vi "W7X1DPut_Reduced.vi"(4 "dimensions":i64[](array[numeric])=[1428413878000000000, -1], 7 "Unit":string="s", 9 "values":T1(array[cluster]), 10 "SigJSONbuffer":string, 11 "SigLabel":string="MTau") -> (0 "Parlog error out":errorcluster, 1 "file path written":string)   [LabVIEW 2014]
uses:
  <vilib>/httpClient/POSTBuffer.vi
  <vilib>/httpClient/LabVIEWHTTPClient.lvlib
panel:
  in  "?":T2
  out "JSON string":string
  out "body":string
  out "headers":string
  out "body Parlog":string
  out "headers parms":string
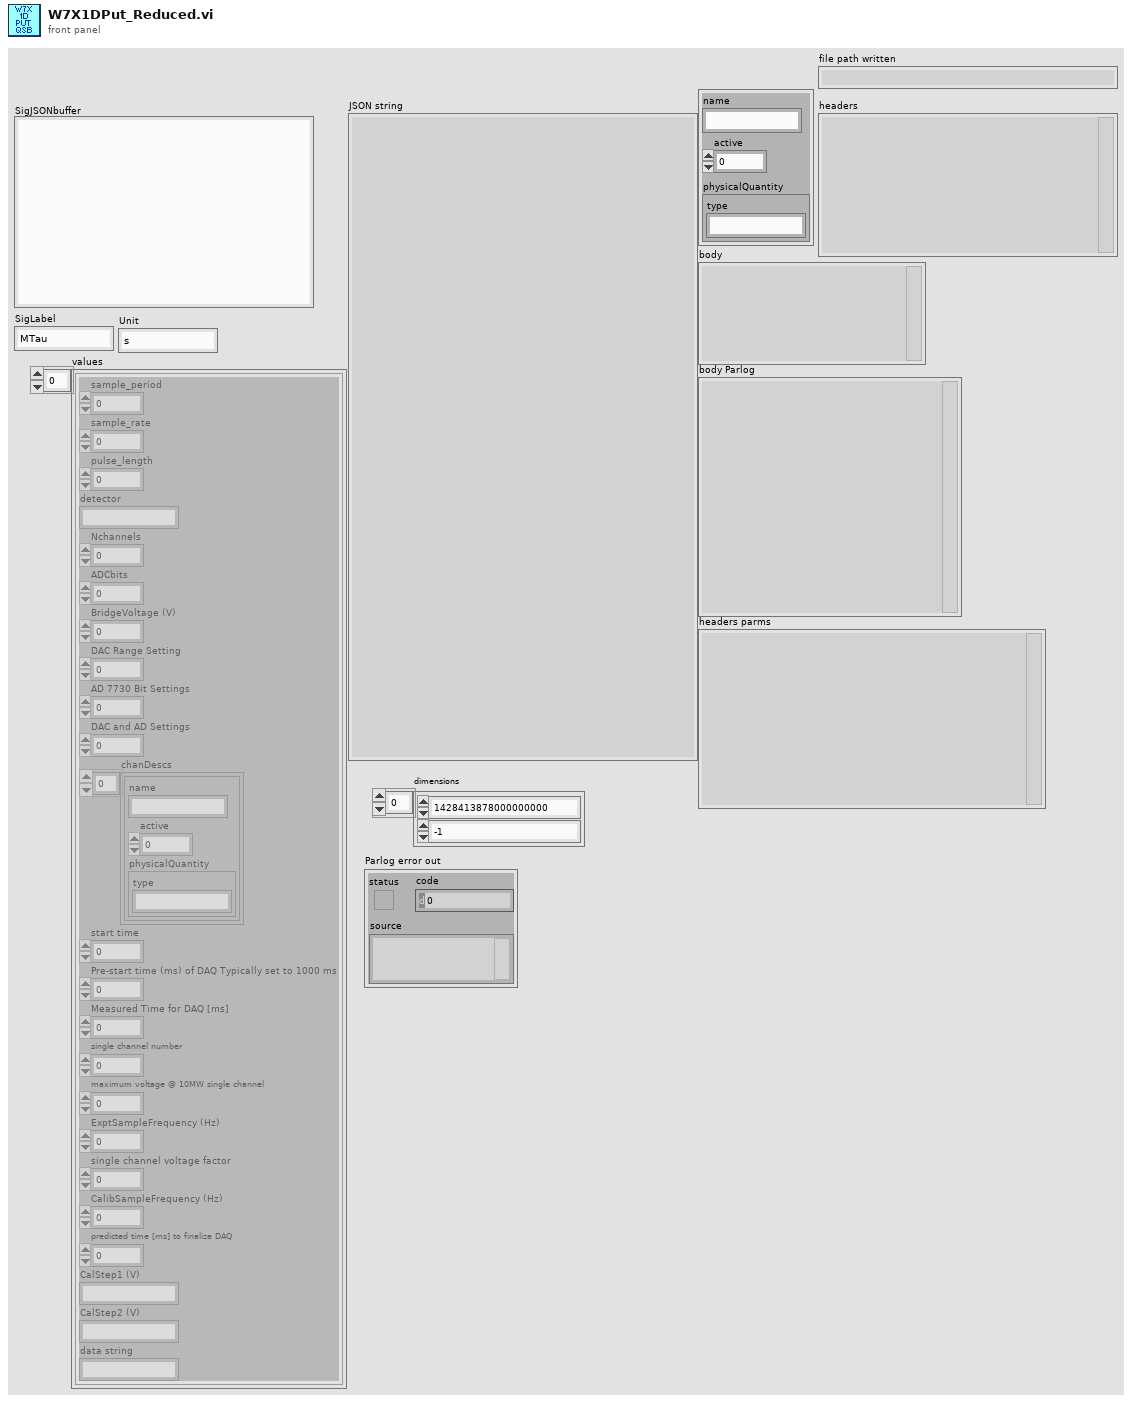
[diagram p1: front panel]
types:
  T1 = cluster{"sample_period":dbl, "sample_rate":dbl, "pulse_length":dbl, "detector":string, "Nchannels":i16, "ADCbits":i16, "BridgeVoltage (V)":sgl, "DAC Range Setting":u8, "AD 7730 Bit Settings":i32, "DAC and AD Settings":i32, "chanDescs":cluster{"name":string, "active":i32, "physicalQuantity":cluster{"type":string}}[], "start time":i64, "Pre-start time (ms) of DAQ Typically set to 1000 ms":i32, "Measured Time for DAQ [ms] ":u32, "single channel number":i64, "maximum voltage @ 10MW single channel":dbl, "ExptSampleFrequency (Hz)":sgl, "single channel voltage factor":dbl, "CalibSampleFrequency (Hz)":sgl, "predicted time [ms] to finalize DAQ":dbl, "CalStep1 (V)":string, "CalStep2 (V)":string, "data string":string}[]
  T2 = cluster{"name":string, "active":i32, "physicalQuantity":cluster{"type":string}}
  T3 = cluster{"sample_period":dbl, "sample_rate":dbl, "pulse_length":dbl, "detector":string, "Nchannels":i16, "ADCbits":i16, "BridgeVoltage (V)":sgl, "DAC Range Setting":u8, "AD 7730 Bit Settings":i32, "DAC and AD Settings":i32, "chanDescs":cluster{"name":string, "active":i32, "physicalQuantity":cluster{"type":string}}[], "start time":i64, "Pre-start time (ms) of DAQ Typically set to 1000 ms":i32, "Measured Time for DAQ [ms] ":u32, "single channel number":i64, "maximum voltage @ 10MW single channel":dbl, "ExptSampleFrequency (Hz)":sgl, "single channel voltage factor":dbl, "CalibSampleFrequency (Hz)":sgl, "predicted time [ms] to finalize DAQ":dbl, "CalStep1 (V)":string, "CalStep2 (V)":string, "data string":string}
  T4 = cluster{"name":string, "active":i32, "physicalQuantity":cluster{"type":string}}[]
  T5 = typedef "LabVIEWHTTPClient.lvlib/ClientHandle.ctl" = refnum<k1>
  T6 = cluster{"label":string, "values":cluster{"sample_period":dbl, "sample_rate":dbl, "pulse_length":dbl, "detector":string, "Nchannels":i16, "ADCbits":i16, "BridgeVoltage (V)":sgl, "DAC Range Setting":u8, "AD 7730 Bit Settings":i32, "DAC and AD Settings":i32, "chanDescs":cluster{"name":string, "active":i32, "physicalQuantity":cluster{"type":string}}[], "start time":i64, "Pre-start time (ms) of DAQ Typically set to 1000 ms":i32, "Measured Time for DAQ [ms] ":u32, "single channel number":i64, "maximum voltage @ 10MW single channel":dbl, "ExptSampleFrequency (Hz)":sgl, "single channel voltage factor":dbl, "CalibSampleFrequency (Hz)":sgl, "predicted time [ms] to finalize DAQ":dbl, "CalStep1 (V)":string, "CalStep2 (V)":string, "data string":string}[], "dimensions":i64[]}
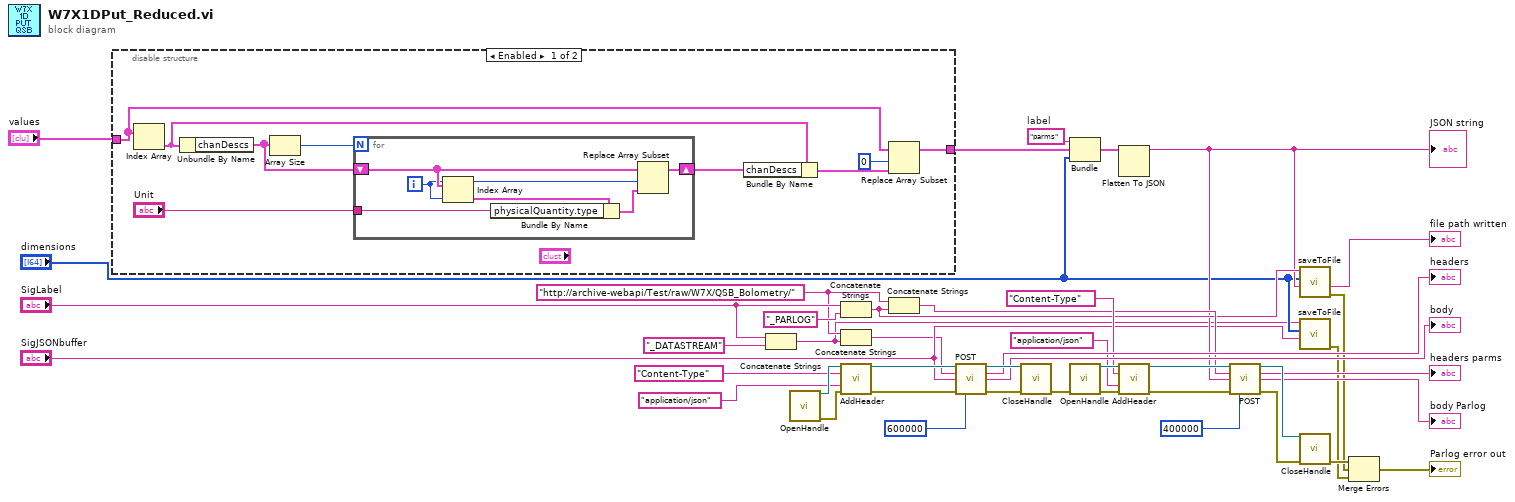
[diagram p0: block diagram]
diagram:
  w31 = "parms"  # label
  w6 = "http://archive-webapi/Test/raw/W7X/QSB_Bolometry/" ("url")
  n1 = disable-structure shown="Enabled" {
    disable-tunnel: "values" -> [w52 w59]
    disable-tunnel: [w51 w59] -> w29
    frame Enabled {
      n2 = Index Array(array=w52) -> (element=w49:T3)  [unwired: 1 in]
      n3 = Unbundle By Name(w49) -> ("chanDescs"=w45:T4)
      n4 = Array Size(array=w45) -> (size(s)=w44:i32)
      n5 = for {
        N: w44 -> [_]
        tunnel: "Unit" -> [w58]
        shift-right: [w54] -> w46
        shift-left: w45 -> [w56]
        i -> [w53]
        n6 = Index Array(array=w56, index=w53) -> (element=w57:T2)
        n7 = Bundle By Name(cluster=w57, "physicalQuantity.type"=w58) -> (w55:T2)
        n8 = Replace Array Subset(array=w56, new element=w55, index=w53) -> (w54:T4)
      }
      n9 = Bundle By Name(cluster=w49, "chanDescs"=w46) -> (w48:T3)
      n10 = Replace Array Subset(array=w52, new element=w48, index=0) -> (w51:T1)
    }
    frame Disabled {
    }
  }
  n11 = Concatenate Strings("SigLabel", "_DATASTREAM" ("string")) -> (w5:string)
  n12 = call <vilib>:"OpenHandle.vi"() -> ("client handle out"=w40:T5, "error out"=w39:errorcluster)  [unwired: 14 in]
  n13 = Concatenate Strings("SigLabel", "_PARLOG" ("replace string (\"\")")) -> (w11:string)
  n14 = Concatenate Strings(w6, w5) -> (w7:string)
  n15 = call <vilib>:"AddHeader.vi"("client handle"=w40, "header"="Content-Type", "value"="application/json", "error in (no error)"=w39) -> ("client handle out"=w38:T5, "error out"=w37:errorcluster)  [unwired: 10 in]
  n16 = Concatenate Strings(w6, w11) -> (w12:string)
  n17 = call-poly <vilib>:"POST.vi"("client handle"=w38, "url"=w7, "buffer"="SigJSONbuffer", "error in (no error)"=w37, "timeout (10000)"=600000) -> ("client handle out"=w43:T5, "headers"=→"headers":string, "body"=→"body":string, "error out"=w42:errorcluster)  [unwired: 7 in]
  n18 = call <vilib>:"CloseHandle.vi"("client handle"=w43, "error in (no error)"=w42) -> ("error out"=w4:errorcluster)  [unwired: 13 in]
  n19 = Bundle("label"=w31, "values"=w29, "dimensions"="dimensions") -> (w30:T6)  [unwired: 1 in]
  n20 = call <vilib>:"OpenHandle.vi"("error in (no error)"=w4) -> ("client handle out"=w25:T5, "error out"=w24:errorcluster)  [unwired: 13 in]
  n21 = Flatten To JSON(anything=w30) -> (JSON string=w10:string)  [unwired: 2 in, 1 out]
  "JSON string" <- w10
  n22 = call <vilib>:"AddHeader.vi"("client handle"=w25, "header"="Content-Type", "value"="application/json", "error in (no error)"=w24) -> ("client handle out"=w23:T5, "error out"=w22:errorcluster)  [unwired: 10 in]
  n23 = call-poly <vilib>:"POST.vi"("client handle"=w23, "url"=w12, "buffer"=w10, "error in (no error)"=w22, "timeout (10000)"=400000) -> ("client handle out"=w28:T5, "headers"=→"headers parms":string, "body"=→"body Parlog":string, "error out"=w27:errorcluster)  [unwired: 7 in]
  n24 = call "saveToFile.vi"("SigJSONbuffer"=w10, "dimensions"="dimensions", "String"=w11) -> ("error out"=w13:errorcluster, "resulting string"=→"file path written":string)  [unwired: 7 in]
  n25 = call "saveToFile.vi"("SigJSONbuffer"="SigJSONbuffer", "dimensions"="dimensions", "String"=w5) -> ("error out"=w3:errorcluster)  [unwired: 7 in, 1 out]
  n26 = call <vilib>:"CloseHandle.vi"("client handle"=w28, "error in (no error)"=w27) -> ("error out"=w17:errorcluster)  [unwired: 13 in]
  n27 = Merge Errors(w17, w13, w3) -> (→"Parlog error out":errorcluster)
